vi "Ramp.vi"(1 "Target Value":dbl, 2 "Ramp Time":dbl, 3 "Inital Value":dbl, 4 "reint":bool) -> (8 "Ramped  Value":dbl)   [LabVIEW 2018]
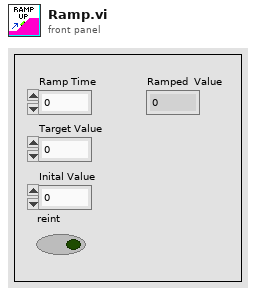
[diagram p1: front panel]
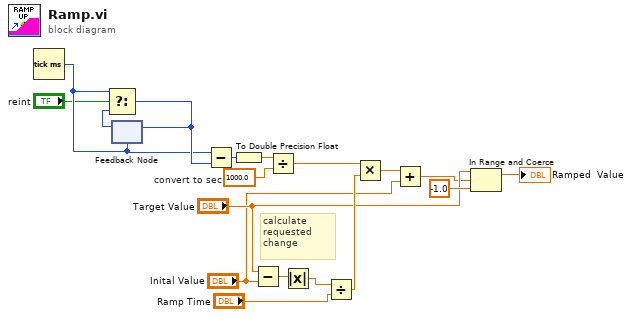
[diagram p0: block diagram]
diagram:
  w12 = 1000.0  # convert to sec
  # "calculate requested\nchange"
  n1 = Tick Count (ms)() -> (millisecond timer value=w16:u32)
  n2 = feedback #1(w16) -> (w18:u32)
  n3 = Select(t=w16, s="reint", f=w18) -> (s? t:f=w17:u32)
  n4 = feedback-in #1(w17) -> ()
  n5 = Subtract(x=w16, y=w17) -> (x-y=w14:u32)
  n6 = To Double Precision Float(number=w14) -> (double precision float=w13:dbl)
  n7 = Subtract(x="Target Value", y="Inital Value") -> (x-y=w5:dbl)
  n8 = Divide(x=w13, y=w12) -> (x/y=w11:dbl)
  n9 = Absolute Value(x=w5) -> (abs(x)=w4:dbl)
  n10 = Divide(x=w4, y="Ramp Time") -> (x/y=w9:dbl)
  n11 = Multiply(x=w11, y=w9) -> (x*y=w3:dbl)
  n12 = Add(x=w3, y="Inital Value") -> (x+y=w2:dbl)
  n13 = In Range and Coerce(upper limit="Target Value", x=w2, lower limit=-1.0) -> (coerced(x)=→"Ramped  Value":dbl)  [unwired: 1 out]
